vi "ESP300Write.vi"(4 "error in (no error)":errorcluster, 5 "Command":string, 6 "ESP300 Axis":string, 7 "ESP300 Address":string) -> (0 "error out":errorcluster)   [LabVIEW 2010]
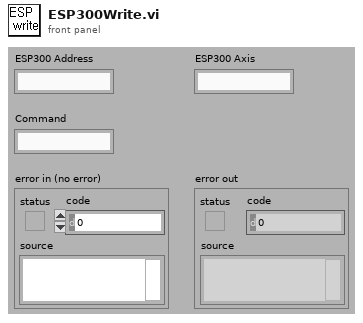
[diagram p1: front panel]
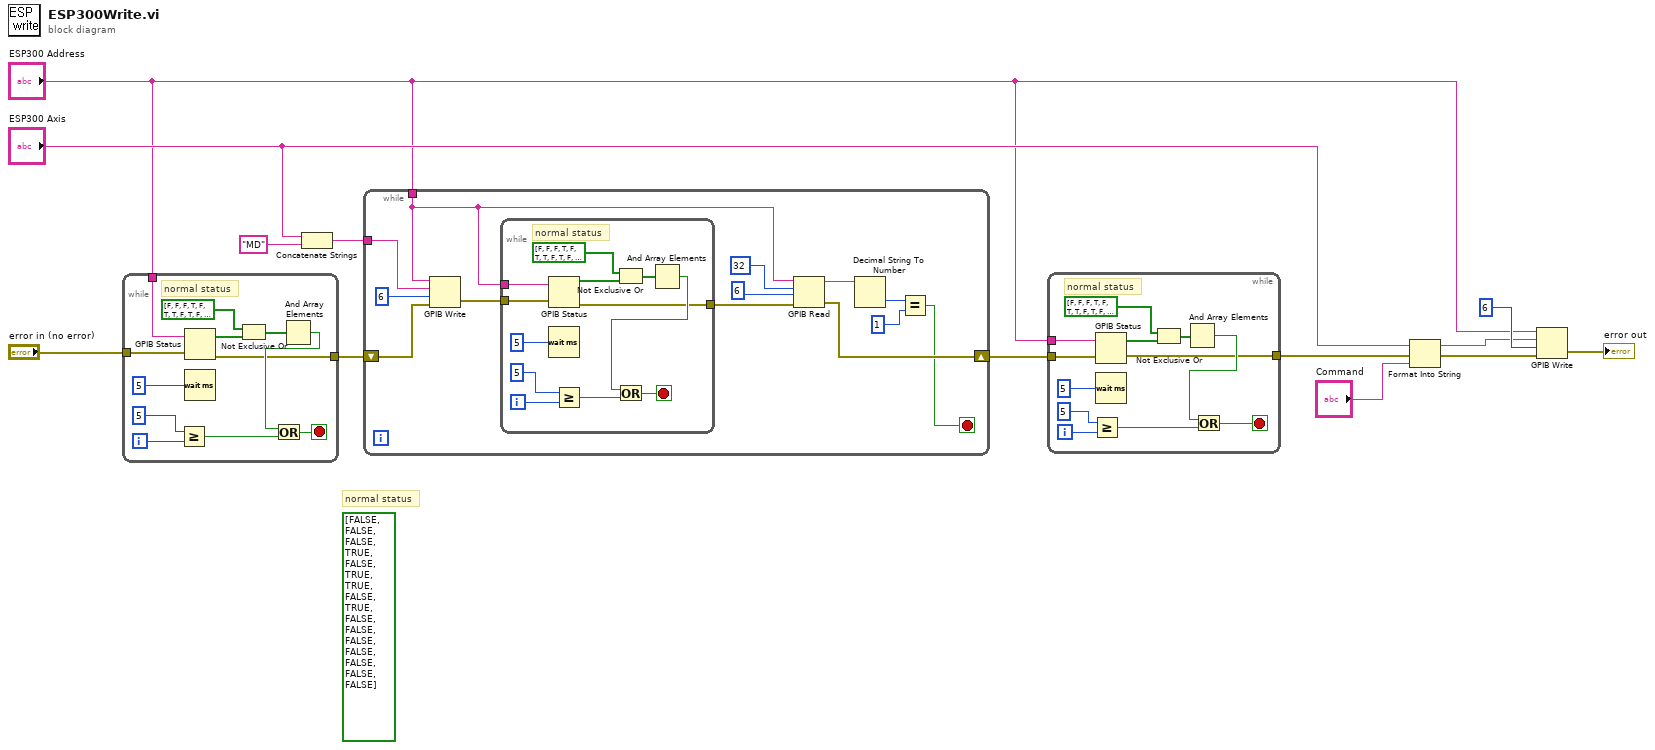
[diagram p0: block diagram]
diagram:
  (unwired) bool[] [FALSE, FALSE, FALSE, TRUE, FALSE, TRUE, TRUE, FALSE, TRUE, FALSE, FALSE, FALSE, FALSE, FALSE, FALSE, FALSE] ("status 2")
  # "normal status"
  n1 = while {
    tunnel: "error in (no error)" -> [w25]
    tunnel: [w15] -> w4
    tunnel: "ESP300 Address" -> [w14]
    i -> [w24]
    stop <- w21 stop-if-true
    # "normal status"
    n2 = Greater Or Equal?(x=5, y=w24) -> (x >= y?=w22:bool)
    n3 = GPIB Status(0:w14, 1:w25) -> (2:w19:bool[], 5:w15:errorcluster)  [unwired: 2 out]
    n4 = Wait (ms)(milliseconds to wait=u32 5) -> ()  [unwired: 1 out]
    n5 = Not Exclusive Or(1:w19, 2:bool[] [FALSE, FALSE, FALSE, TRUE, FALSE, TRUE, TRUE, FALSE, TRUE, FALSE, FALSE, FALSE, FALSE, FALSE, FALSE, FALSE] ("status 2")) -> (0:w18:bool[])
    n6 = And Array Elements(Boolean array=w18) -> (logical AND=w17:bool)
    n7 = Or(x=w17, y=w22) -> (x .or. y?=w21:bool)
  }
  n8 = Concatenate Strings("ESP300 Axis", "MD" ("string")) -> (w10:string)
  n9 = while {
    tunnel: w10 -> [w38]
    shift-right: [w34] -> w3
    shift-left: w4 -> [w36]
    tunnel: "ESP300 Address" -> [w26]
    stop <- w30 stop-if-true
    n10 = GPIB Write(0:w26, 1:w38, 2:i16 6 ("mode (0)"), 3:w36) -> (6:w28:errorcluster)  [unwired: 1 in, 1 out]
    n11 = while {
      tunnel: w28 -> [w50]
      tunnel: [w40] -> w27
      tunnel: w26 -> [w39]
      i -> [w49]
      stop <- w46 stop-if-true
      # "normal status"
      n12 = GPIB Status(0:w39, 1:w50) -> (2:w44:bool[], 5:w40:errorcluster)  [unwired: 2 out]
      n13 = Wait (ms)(milliseconds to wait=u32 5) -> ()  [unwired: 1 out]
      n14 = Greater Or Equal?(x=5, y=w49) -> (x >= y?=w47:bool)
      n15 = Not Exclusive Or(1:w44, 2:bool[] [FALSE, FALSE, FALSE, TRUE, FALSE, TRUE, TRUE, FALSE, TRUE, FALSE, FALSE, FALSE, FALSE, FALSE, FALSE, FALSE] ("status 2")) -> (0:w43:bool[])
      n16 = And Array Elements(Boolean array=w43) -> (logical AND=w42:bool)
      n17 = Or(x=w42, y=w47) -> (x .or. y?=w46:bool)
    }
    n18 = GPIB Read(0:w26, 1:32 ("byte count"), 2:i16 6 ("mode (0)"), 3:w27) -> (5:w33:string, 7:w34:errorcluster)  [unwired: 1 in, 1 out]
    n19 = Decimal String To Number(string=w33) -> (number=w32:i32)  [unwired: 2 in, 1 out]
    n20 = Equal?(x=w32, y=1) -> (x = y?=w30:bool)
  }
  n21 = while {
    tunnel: w3 -> [w62]
    tunnel: [w52] -> w2
    tunnel: "ESP300 Address" -> [w51]
    i -> [w61]
    stop <- w58 stop-if-true
    # "normal status"
    n22 = Greater Or Equal?(x=5, y=w61) -> (x >= y?=w59:bool)
    n23 = GPIB Status(0:w51, 1:w62) -> (2:w56:bool[], 5:w52:errorcluster)  [unwired: 2 out]
    n24 = Wait (ms)(milliseconds to wait=u32 5) -> ()  [unwired: 1 out]
    n25 = Not Exclusive Or(1:w56, 2:bool[] [FALSE, FALSE, FALSE, TRUE, FALSE, TRUE, TRUE, FALSE, TRUE, FALSE, FALSE, FALSE, FALSE, FALSE, FALSE, FALSE] ("status 2")) -> (0:w55:bool[])
    n26 = And Array Elements(Boolean array=w55) -> (logical AND=w54:bool)
    n27 = Or(x=w54, y=w59) -> (x .or. y?=w58:bool)
  }
  n28 = Format Into String(initial string="ESP300 Axis", error in=w2, "Command") -> (resulting string=w12:string, error out=w8:errorcluster)  [unwired: 1 in]
  n29 = GPIB Write(0:"ESP300 Address", 1:w12, 2:i16 6 ("mode (0)"), 3:w8) -> (6:→"error out":errorcluster)  [unwired: 1 in, 1 out]
